vi "HowTo.vi"() -> ()   [LabVIEW 2017]
panel:
  in  "OK":bool
  out "HowTo":string
  # "Como Jogar?"
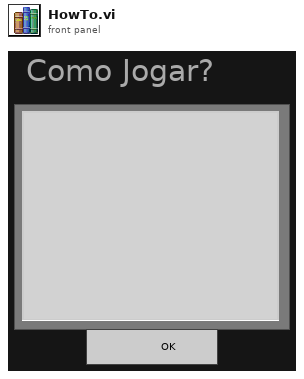
[diagram p1: front panel]
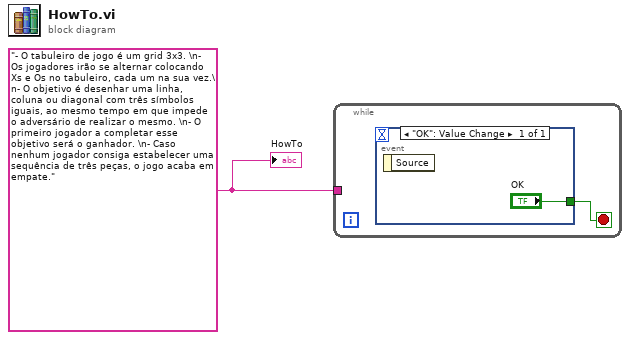
[diagram p0: block diagram]
diagram:
  w1 = "- O tabuleiro de jogo é um grid 3x3. \n- Os jogadores irão se alternar colocando Xs e Os no tabuleiro, cada um na sua vez.\n- O objetivo é desenhar uma linha, coluna ou diagonal com três símbolos iguais, ao mesmo tempo em que impede o adversário de realizar o mesmo. \n- O primeiro jogador a completar esse objetivo será o ganhador. \n- Caso nenhum jogador consiga estabelecer uma sequência de três peças, o jogo acaba em empate."
  n1 = while {
    tunnel: w1 -> [_]
    stop <- w2 stop-if-true
    n2 = event shown="[0] \"OK\": Value Change" {
      selector: _ -> [_]
      dyn-events: _ -> [_]
      timeout: _ -> [_]
      tunnel: ["OK"] -> w2
      event "OK": Value Change {
        n3 = event-data() -> ()  [unwired: 1 in, 1 out]
      }
    }
  }
  "HowTo" <- w1
